vi "get_ID.vi"(8 "error in (no error)":errorcluster, 11 "LakeShore336 in":refnum<class "Lakeshore_336.lvclass">) -> (0 "error out":errorcluster, 2 "ID from Instrument":string, 3 "LakeShore336 out":refnum<class "Lakeshore_336.lvclass">)   [LabVIEW 2018, in "Lakeshore_336.lvclass"]
doc: "the vi reads the ID from the instrument"
uses:
  Lakeshore_336.lvclass
  instrument.lvclass
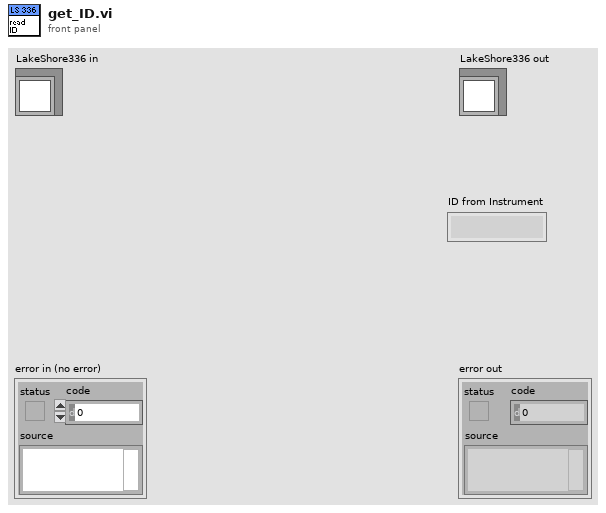
[diagram p1: front panel]
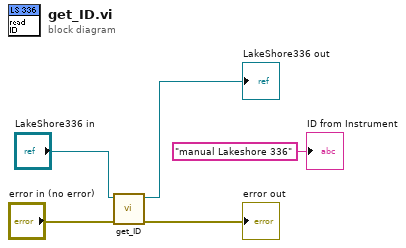
[diagram p0: block diagram]
diagram:
  n1 = call-parent "get_ID.vi"("error in (no error)"="error in (no error)", "instrument in"="LakeShore336 in") -> ("error out"=→"error out":errorcluster, "instrument out"=→"LakeShore336 out":refnum<class "Lakeshore_336.lvclass">)  [unwired: 7 in, 1 out]
  "ID from Instrument" <- "manual Lakeshore 336" ("ID from Instrument")
